vi "SteeringAssist.vi"(8 "Gain":dbl, 9 "Steering Input":i32, 11 "Drive Input":u16) -> (3 "Drive Output":u16)   [LabVIEW 2013, in "ProcessorHelperFunctions.lvlib"]
uses:
  ProcessorHelperFunctions.lvlib
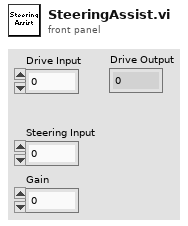
[diagram p1: front panel]
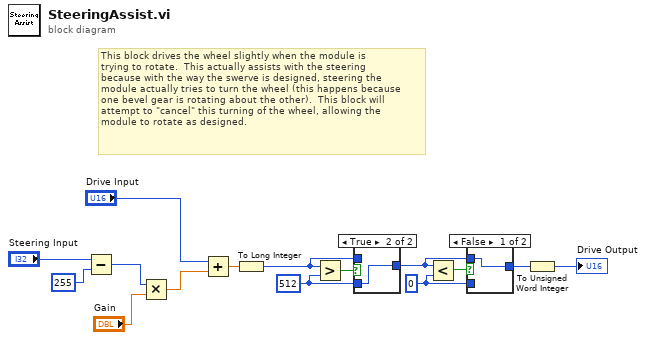
[diagram p0: block diagram]
diagram:
  w11 = u16 0 ("y")
  w10 = u16 512 ("y")
  # "This block drives the wheel slightly when the module is\ntrying to rotate.  This actually assists with the steering\nbecause with the way the swerve is designed, steering the\nmodule actually tries to turn the wheel (this happens because\none bevel gear is rotating about the other).  This block will\nattempt to \"cancel\" this turning of the wheel, allowing the\nmodule to rotate as designed."
  n1 = Subtract(x="Steering Input", y=255) -> (x-y=w2:i32)
  n2 = Multiply(x=w2, y="Gain") -> (x*y=w13:dbl)
  n3 = Add(x="Drive Input", y=w13) -> (x+y=w7:dbl)
  n4 = To Long Integer(number=w7) -> (32bit integer=w6:i32)
  n5 = Greater?(x=w6, y=w10) -> (0:w9:bool)
  n6 = case shown="True" w9 {
    tunnel: w10 -> [_ w17]
    tunnel: w6 -> [w16 _]
    tunnel: [w16 w17] -> w12
    frame False {
    }
    frame True {
    }
  }
  n7 = Less?(x=w12, y=w11) -> (x < y?=w8:bool)
  n8 = case shown="False" w8 {
    tunnel: w11 -> [_ w19]
    tunnel: w12 -> [w18 _]
    tunnel: [w18 w19] -> w5
    frame False {
    }
    frame True {
    }
  }
  n9 = To Unsigned Word Integer(number=w5) -> (unsigned 16bit integer=→"Drive Output":u16)
